vi "Channel Monitor (DAQmx).vi"() -> ()   [LabVIEW 2009]
doc: "This example shows how to use the Channel Monitor XControl with DAQmx devices. The channel names from the \nDAQmx channels will automatically be used in the Channel Monitor.\n\nSome things to try:\n-To view the actual time domain signal, you can click on an associated button to launch a display.\n-Expand the XControl vertical to add more visible rows.\n-In edit time, right-click the XControl and select \"Change Level Color\" to change the color of the bars."
uses:
  user.lib/Channel Monitor/Channel Monitor.xctl
  <vilib>/Utility/error.llb/DialogType.ctl
  <vilib>/DAQmx/configure/timing.llb/DAQmx Timing (Sample Clock).vi
  <vilib>/DAQmx/create/channels.llb/DAQmx Create Channel (AI-Voltage-Basic).vi
  <vilib>/DAQmx/read.llb/DAQmx Read (Analog 1D Wfm NChan NSamp).vi
  Program Files/National Instruments/LabVIEW 2009/resource/objmgr/daqmx.rc
panel:
  out "Channel Monitor":waveform(dbl)[](xcontrol)
  in  "Samples to Read":i32=1000
  in  "Physical Channel":tag="cDAQ2Mod1/ai0:3, cDAQ2Mod2/ai0:3, cDAQ2Mod3/ai0:3"
  in  "Minimum Value":dbl=-5.0 format="%0.2f"
  in  "Maximum Value":dbl=5.0 format="%0.2f"
  in  "stop":bool
  in  "Sample Rate":dbl=10000.0 caption="Sample Rate (Hz)" format="%0.2f"
  # "This example shows how to use the Channel Monitor XControl with DAQmx devices.  The channel names from the \nDAQmx channels will automatically be used in the Channel Monitor.\n\nSome things to try:\n-To view the actual time domain signal, you can click on an associated button to launch a display.\n-Expand the XControl vertical to add more visible rows.\n-In edit time, right-click the XControl and select \"Change Level Color\" to change the color of the bars."
  # "Channel Parameters"
  # "Timing Parameters"
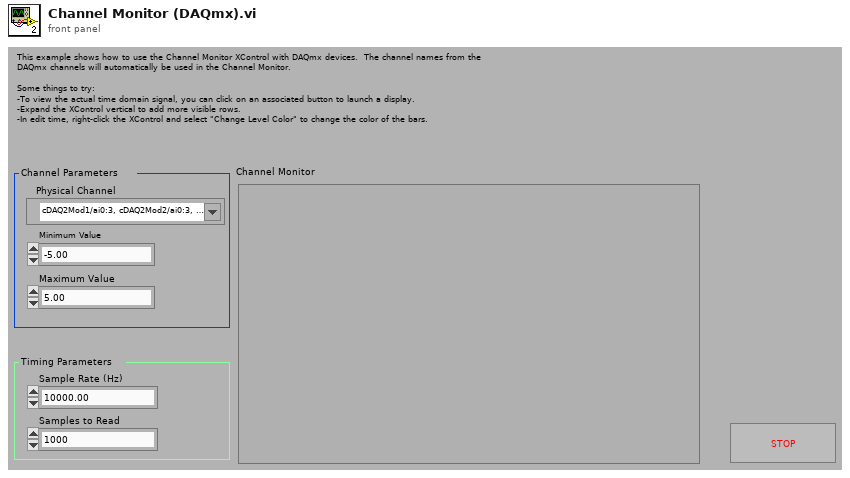
[diagram p1: front panel]
types:
  T1 = typedef "DialogType.ctl" = u16
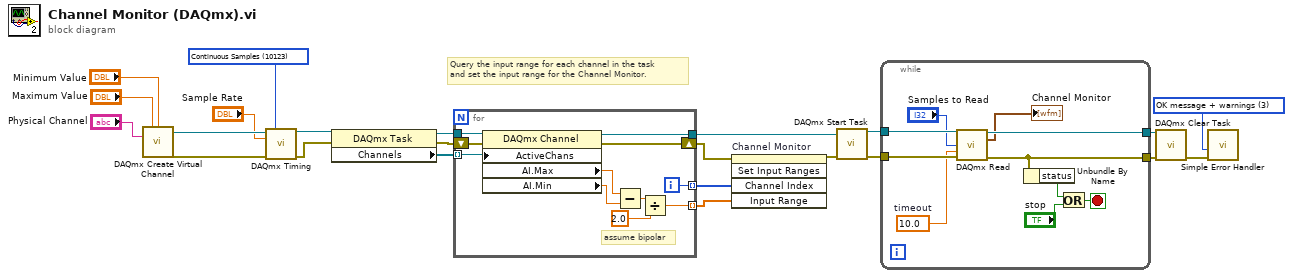
[diagram p0: block diagram]
diagram:
  w11 = T1 3 items=["no dialog", "OK message", "continue or stop message", "OK message + warnings", "continue/stop + warnings"] ("type of dialog (OK msg:1)")
  w14 = 10123 items=["Finite Samples"=10178, "Continuous Samples"=10123] ("sample mode")
  # "Query the input range for each channel in the task\nand set the input range for the Channel Monitor."
  n1 = call-poly <vilib>:"DAQmx Create Virtual Channel.vi"("maximum value"="Maximum Value", "minimum value"="Minimum Value", "physical channels"="Physical Channel") -> ("task out"=w18:refnum<k21>, "error out"=w21:errorcluster)  [unwired: 11 in]
  n2 = call-poly <vilib>:"DAQmx Timing.vi"("task/channels in"=w18, "sample mode"=w14, "rate"="Sample Rate", "error in"=w21) -> ("task out"=w6:refnum<k21>, "error out"=w5:errorcluster)  [unwired: 10 in]
  n3 = property class="DAQmx Task"(reference=w6, error in=w5) -> (reference out=w9:refnum<k21>, error out=w7:errorcluster, "Channels"=w8:refnum<k21>[])
  n4 = for {
    tunnel: w9 -> [w31]
    tunnel: w8 -> [w30] mode=indexing
    shift-right: [w28] -> w4
    shift-left: w7 -> [w29]
    tunnel: [w26] -> w3
    tunnel: [w25] -> w2 mode=indexing
    tunnel: [w24] -> w1 mode=indexing
    i -> [w24]
    # "assume bipolar"
    n5 = property class="DAQmx Channel"(reference=w31, error in=w29, "ActiveChans"=w30) -> (reference out=w26:refnum<k21>, error out=w28:errorcluster, "AI.Max"=w27:dbl, "AI.Min"=w34:dbl)
    n6 = Subtract(x=w27, y=w34) -> (x-y=w33:dbl)
    n7 = Divide(x=w33, y=2.0) -> (x/y=w25:dbl)
  }
  n8 = invoke on="Channel Monitor" class="Channel Monitor (strict)" method="Set Input Ranges"(error in=w4, "Channel Index"=w1, "Input Range"=w2) -> (error out=w10:errorcluster)  [unwired: 2 in, 4 out]
  n9 = call <vilib>:"DAQmx Start Task.vi"("task/channels in"=w3, "error in"=w10) -> ("task out"=w17:refnum<k21>, "error out"=w20:errorcluster)  [unwired: 12 in]
  n10 = while {
    tunnel: w20 -> [w44]
    tunnel: w17 -> [w43]
    tunnel: [w42] -> w16
    tunnel: [w41] -> w13
    stop <- w39 stop-if-true
    w37 = 10.0  # timeout
    n11 = call-poly <vilib>:"DAQmx Read.vi"("task/channels in"=w43, "number of samples per channel"="Samples to Read", "timeout"=w37, "error in"=w44) -> ("task out"=w42:refnum<k21>, "data"=→"Channel Monitor":waveform(dbl)[], "error out"=w41:errorcluster)  [unwired: 9 in]
    n12 = Unbundle By Name(w41) -> ("status"=w40:bool)
    n13 = Or(x=w40, y="stop") -> (x .or. y?=w39:bool)
  }
  n14 = call <vilib>:"DAQmx Clear Task.vi"("task in"=w16, "error in"=w13) -> ("error out"=w19:errorcluster)  [unwired: 13 in]
  n15 = call <vilib>:"Simple Error Handler.vi"("type of dialog (OK msg:1)"=w11, "error in (no error)"=w19) -> ()  [unwired: 3 in, 5 out]
